vi "Protocol Engine.vi"(8 "error in (no error)":errorcluster, 10 "Settings":T1 {"Compiled"."External Channels"."Channels" format="%.0x"; "Compiled"."External Channels"."Triggers" format="%.0x"}, 11 "State Variables":T14) -> (0 "error out":errorcluster)   [LabVIEW 2019, in "Instrument Addon Engine.lvlib"]
uses:
  Instrument Addon Engine.lvlib
  Types/Engine State Variables.ctl
  <vilib>/NI/NI VeriStand Addon Network Comm/Engine/VeriStand Comm.lvclass
  <vilib>/NI/NIVS Inline Async API/_VS Inline Async API/Process/Process.lvclass
  <vilib>/NI/NIVS Inline Async API/_Data Access Engine/Data Access Engine/Types/Write.DVR.ctl
  <vilib>/NI/NIVS Inline Async API/_Data Access Engine/Access Type Classes/Write/Write.lvclass
  <vilib>/NI/NIVS Inline Async API/_Data Access Engine/Data Access Engine/Types/Read.DVR.ctl
  <vilib>/NI/NIVS Inline Async API/_Data Access Engine/Access Type Classes/Read/Read.lvclass
  <vilib>/NI/NIVS Inline Async API/_Data Access Engine/Data Access Engine/Types/ReadWrite.DVR.ctl
  <vilib>/NI/NIVS Inline Async API/_Data Access Engine/Access Type Classes/ReadWrite/ReadWrite.lvclass
  Types/Commands RT Configuration Cluster.ctl
  Includes/Protocols.lvlibp/Protocol Parent/Protocol Parent.lvclass
  Addon Shared/Types/Compiled Settings.ctl
  Addon Shared/Types/Command Parameters.ctl
  Addon Shared/Types/Linked Channel Cluster.ctl
  Addon Shared/Types/Command Channel Indeces.ctl
  Addon Shared/Types/Command Channel Index.ctl
  Addon Shared/Types/Response RT Configuration Cluster.ctl
  Addon Shared/Types/Response Parameters.ctl
  Addon Shared/Types/Response Wait Type.ctl
  Addon Shared/Types/Message Parameters.ctl
  Addon Shared/Types/Message Generation Type.ctl
  Addon Shared/Types/External Trigger Refs.ctl
  <vilib>/NI VeriStand/Custom Device API/Data Reference.ctl
  Includes/Protections.lvlibp/Parent Protection/Protection.lvclass
  <vilib>/NI/NI VeriStand Addon Network Comm/Engine/VeriStand Comm.lvclass/VeriStand Comm.ctl
  Addon Shared/Types/Buffered RT Instrument Command.ctl
  Includes/Protocols.lvlibp/Protocol Parent/Methods/Read Parameter.ctl
  Addon Shared/Types/Buffered RT Instrument Request.ctl
  <vilib>/NI/NIVS Inline Async API/_VS Inline Async API/Process/Process.lvclass/Process.ctl
  <vilib>/NI/NIVS Inline Async API/_VS Inline Async API/Error Handling Process/SubVIs/Error.ConvertArray.vi
  <vilib>/NI/NI VeriStand Addon Network Comm/Shared/Comm Constants.vi
  <vilib>/NI/AMC/Read Next Message.vi
  <vilib>/NI/Tools/Keyed Array/Index.vi
  <vilib>/NI/AMC/Send Local Message.vi
  Addon Shared/Instrument Addon Shared.lvlib
  <vilib>/NI VeriStand/Custom Device API/Custom Device API.lvlib
  <vilib>/NI/NIVS Inline Async API/_Data Access Engine/Data Access Engine/Data Access Engine.lvclass
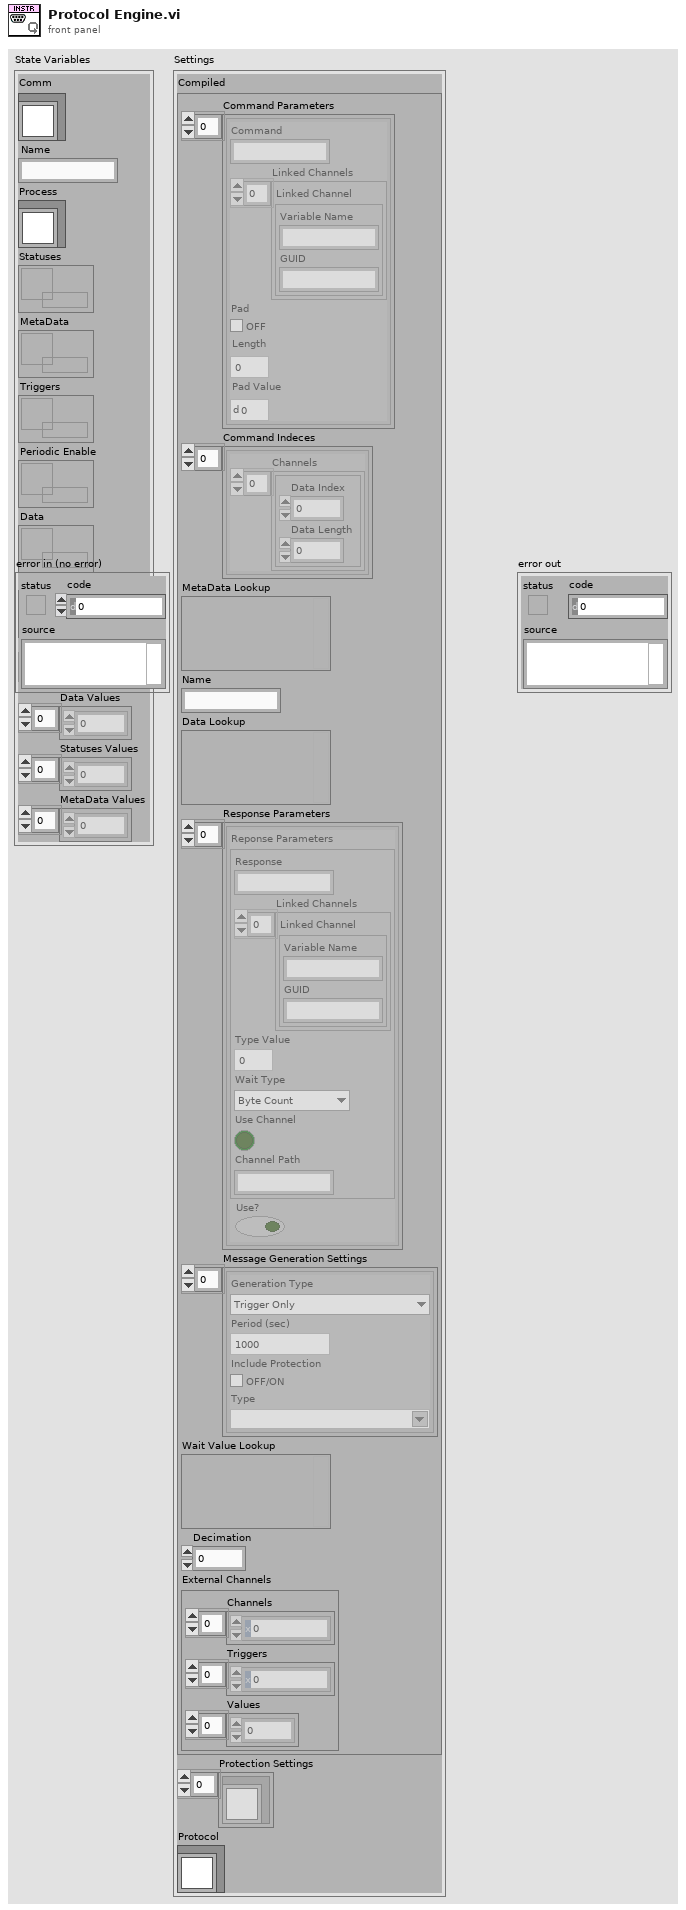
[diagram p1: front panel]
types:
  T1 = typedef "Instrument Addon Engine.lvlib/Commands RT Configuration Cluster.ctl" = cluster{"Compiled":T2, "Protection Settings":refnum<class "Protection.lvclass">[], "Protocol":refnum<class "Protocol Parent.lvclass">}
  T2 = typedef "Instrument Addon Shared.lvlib/Compiled Settings.ctl" = cluster{"Command Parameters":T3[], "Command Indeces":T5[], "MetaData Lookup":variant, "Name":string, "Data Lookup":variant, "Response Parameters":T7[], "Message Generation Settings":T10[], "Wait Value Lookup":variant, "Decimation":u32, "External Channels":T12}
  T3 = typedef "Instrument Addon Shared.lvlib/Command Parameters.ctl" = cluster{"Command":string, "Linked Channels":T4[], "Pad":bool, "Length":u32, "Pad Value":u8}
  T4 = typedef "Instrument Addon Shared.lvlib/Linked Channel Cluster.ctl" = cluster{"Variable Name":string, "GUID":string}
  T5 = typedef "Instrument Addon Shared.lvlib/Command Channel Indeces.ctl" = cluster{"Channels":T6[]}
  T6 = typedef "Instrument Addon Shared.lvlib/Command Channel Index.ctl" = cluster{"Data Index":i32, "Data Length":i32}
  T7 = typedef "Instrument Addon Shared.lvlib/Response RT Configuration Cluster.ctl" = cluster{"Reponse Parameters":T8, "Use?":bool}
  T8 = typedef "Instrument Addon Shared.lvlib/Response Parameters.ctl" = cluster{"Response":string, "Linked Channels":T4[], "Type Value":dbl, "Wait Type":T9, "Use Channel":bool, "Channel Path":string}
  T9 = typedef "Instrument Addon Shared.lvlib/Response Wait Type.ctl" = enum16{"Byte Count", "Wait sec"}
  T10 = typedef "Instrument Addon Shared.lvlib/Message Parameters.ctl" = cluster{"Generation Type":T11, "Period":dbl, "Include Protection":bool, "Type":string}
  T11 = typedef "Instrument Addon Shared.lvlib/Message Generation Type.ctl" = enum16{"Trigger Only", "Periodic & Trigger", "Value Change & Trigger"}
  T12 = typedef "Instrument Addon Shared.lvlib/External Trigger Refs.ctl" = cluster{"Channels":T13[], "Triggers":T13[], "Values":dbl[]}
  T13 = typedef "Custom Device API.lvlib/Data Reference.ctl" = i32
  T14 = typedef "Instrument Addon Engine.lvlib/Engine State Variables.ctl" = cluster{"Comm":refnum<class "VeriStand Comm.lvclass">, "Name":string, "Process":refnum<class "Process.lvclass">, "Statuses":T15, "MetaData":T16, "Triggers":T17, "Periodic Enable":T16, "Data":T15, "Wait":T16, "Wait Values":dbl[], "Data Values":dbl[], "Statuses Values":dbl[], "MetaData Values":dbl[]}
  T15 = typedef "Data Access Engine.lvlib/Data Access Engine.lvclass/Write.DVR.ctl" = refnum<data-value>
  T16 = typedef "Data Access Engine.lvlib/Data Access Engine.lvclass/Read.DVR.ctl" = refnum<data-value>
  T17 = typedef "Data Access Engine.lvlib/Data Access Engine.lvclass/ReadWrite.DVR.ctl" = refnum<data-value>
  T18 = typedef "Instrument Addon Shared.lvlib/Buffered RT Instrument Command.ctl" = cluster{"Command":string, "Response Expected?":bool, "Wait Type":T9, "Wait Value":dbl}
  T19 = typedef "Instrument Addon Shared.lvlib/Buffered RT Instrument Request.ctl" = cluster{"Response":string, "Error":errorcluster}
  T20 = typedef "Protocols.lvlibp/Protocol Parent.lvclass/Read Parameter.ctl" = cluster{"Wait Type":enum16{"Byte Count", "Wait sec"}, "Wait Value":dbl}
  T21 = typedef "NI VeriStand Addon Network Comm.lvlib/VeriStand Comm.lvclass/Response Information.ctl" = cluster{"response name":string, "responseQ":string}
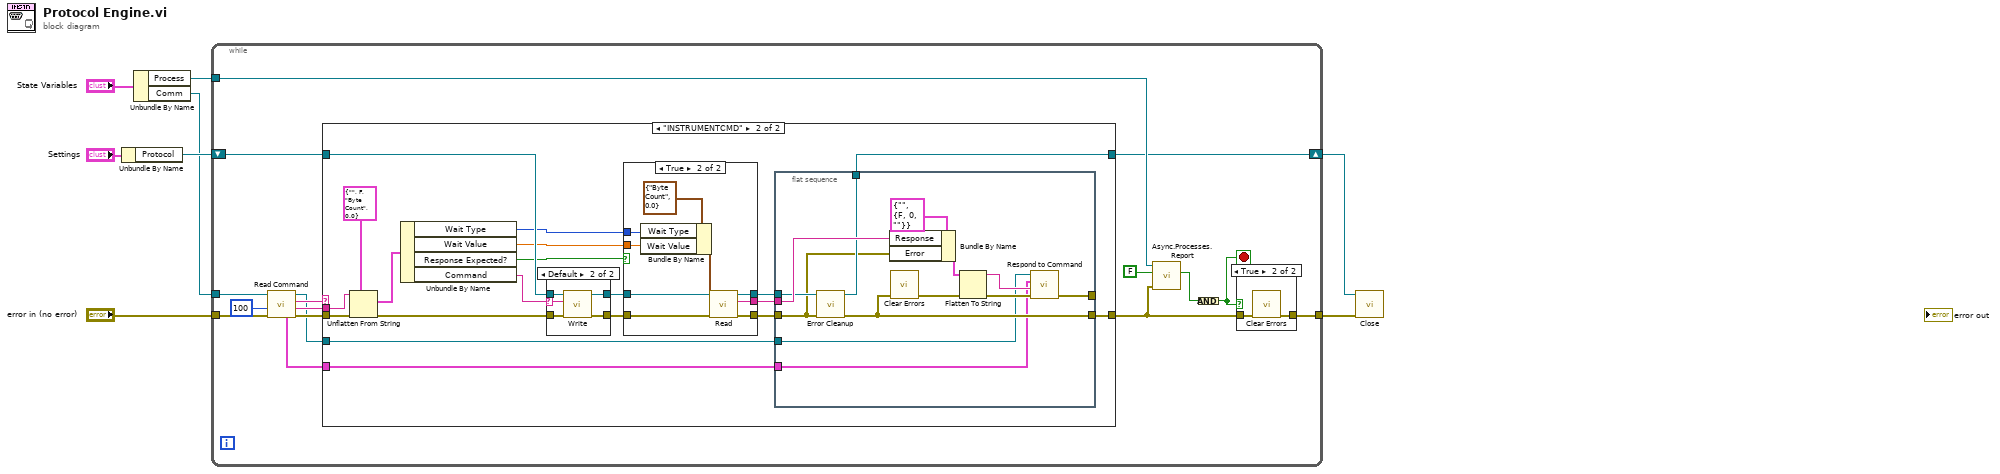
[diagram p0: block diagram]
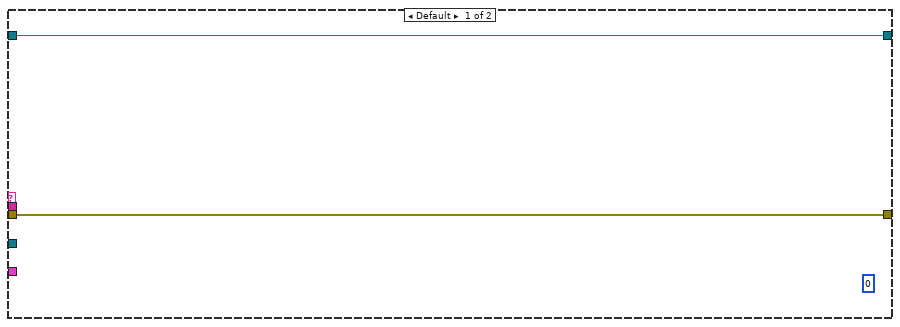
[diagram p2: hidden frame]
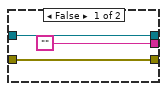
[diagram p4: hidden frame]
diagram:
  n1 = Unbundle By Name("Settings") -> ("Protocol"=w5:refnum<class "Protocol Parent.lvclass">)
  n2 = Unbundle By Name("State Variables") -> ("Process"=w8:refnum<class "Process.lvclass">, "Comm"=w1:refnum<class "VeriStand Comm.lvclass">)
  n3 = while {
    tunnel: "error in (no error)" -> [w16]
    tunnel: [w18] -> w3
    tunnel: w8 -> [w23]
    shift-right: [w20] -> w4
    shift-left: w5 -> [w21]
    tunnel: w1 -> [w10]
    stop <- w19 stop-if-true
    n4 = call <vilib>:"Read Command.vi"("error in (no error)"=w16, "timeout (100 ms)"=100 ("timeout (1 ms)"), "VeriStand Comm in"=w10) -> ("error out"=w11:errorcluster, "message value"=w14:string, "message name"=w13:string, "VeriStand Comm out"=w9:refnum<class "VeriStand Comm.lvclass">, "ResponseInfo"=w15:T21)  [unwired: 3 in, 1 out]
    n5 = case shown="\"INSTRUMENTCMD\"" w13 {
      tunnel: w11 -> [w26 w41]
      tunnel: w14 -> [_ w45]
      tunnel: w21 -> [w25 w43]
      tunnel: [w26 w34] -> w17
      tunnel: w15 -> [_ w28]
      tunnel: [w25 w29] -> w20
      tunnel: w9 -> [_ w27]
      frame Default {
        (unwired) u32 0
      }
      frame "INSTRUMENTCMD" {
        n6 = Unflatten From String(type=T18 {"Command"="", "Response Expected?"=FALSE, "Wait Type"=enum."Byte Count", "Wait Value"=0.0} ("Buffered Command Cluster"), binary string=w45, error in (no error)=w41) -> (value=w38:T18, error out=w40:errorcluster)  [unwired: 2 in, 1 out]
        n7 = Unbundle By Name(w38) -> ("Wait Type"=w33:T9, "Wait Value"=w32:dbl, "Response Expected?"=w37:bool, "Command"=w31:string)
        n8 = case shown="Default" w31 {
          selector: w31 -> [_ w48]
          tunnel: [w46 w52] -> w44
          tunnel: w43 -> [w47 w51]
          tunnel: [w47 w50] -> w42
          tunnel: w40 -> [w46 w49]
          frame "" {
          }
          frame Default {
            n9 = call-dynamic "Write.vi"("error in (no error)"=w49, "String"=w48, "Protocol Parent in"=w51) -> ("error out"=w52:errorcluster, "Protocol Parent out"=w50:refnum<class "Protocol Parent.lvclass">)  [unwired: 7 in]
          }
        }
        n10 = case shown="True" w37 {
          tunnel: w44 -> [w68 w75]
          tunnel: w42 -> [w66 w74]
          tunnel: [w68 w77] -> w36
          tunnel: ["" w76] -> w35
          tunnel: w33 -> [_ w71]
          tunnel: w32 -> [_ w73]
          tunnel: [w66 w72] -> w30
          frame False {
          }
          frame True {
            n11 = Bundle By Name(cluster=T20 {"Wait Type"=enum."Byte Count", "Wait Value"=0.0} ("Read Parameter"), "Wait Type"=w71, "Wait Value"=w73) -> (w69:T20)
            n12 = call-dynamic "Read.vi"("error in (no error)"=w75, "Variant"=w69, "Protocol Parent in"=w74) -> ("error out"=w77:errorcluster, "String"=w76:string, "Protocol Parent out"=w72:refnum<class "Protocol Parent.lvclass">)  [unwired: 6 in]
          }
        }
        n13 = flat-sequence {
          tunnel: w36 -> [w55]
          tunnel: w35 -> [w64]
          tunnel: [w58] -> w34
          tunnel: [w59] -> _
          tunnel: w30 -> [w57]
          tunnel: [w56] -> w29
          tunnel: w28 -> [w54]
          tunnel: w27 -> [w53]
          frame #0 {
            n14 = call-dynamic "Error Cleanup.vi"("error in (no error)"=w55, "Protocol Parent in"=w57) -> ("error out"=w58:errorcluster, "Protocol Parent out"=w56:refnum<class "Protocol Parent.lvclass">)  [unwired: 8 in]
            n15 = Bundle By Name(cluster=T19 {"Response"="", "Error"={"status"=FALSE, "code"=0, "source"=""}}, "Response"=w64, "Error"=w55) -> (w63:T19)
            n16 = call <vilib>:"Clear Errors.vi"("error in (no error)"=w58) -> ("error out"=w62:errorcluster)  [unwired: 5 in, 1 out]
            n17 = Flatten To String(anything=w63, error in (no error)=w62) -> (data string=w60:string, error out=w61:errorcluster)  [unwired: 2 in, 1 out]
            n18 = call <vilib>:"Respond to Command.vi"("error in (no error)"=w61, "message value"=w60, "ResponseInfo"=w54, "VeriStand Comm in"=w53) -> ("error out"=w59:errorcluster)  [unwired: 5 in, 2 out]
          }
        }
      }
    }
    n19 = call <vilib>:"Async.Processes.Report.vi"("Error"=w17, "Stop Async on Error?"=FALSE ("Stop on Error?"), "Process in"=w23) -> ("Stop"=w24:bool)  [unwired: 7 in, 1 out]
    n20 = Compound Arithmetic op=AND(w24) -> (w19:bool)
    n21 = case shown="True" w19 {
      tunnel: w17 -> [w78 w80]
      tunnel: [w78 w79] -> w18
      frame False {
      }
      frame True {
        n22 = call <vilib>:"Clear Errors.vi"("error in (no error)"=w80) -> ("error out"=w79:errorcluster)  [unwired: 5 in, 1 out]
      }
    }
  }
  n23 = call-dynamic "Close.vi"("error in (no error)"=w3, "Protocol Parent in"=w4) -> ()  [unwired: 8 in, 2 out]
